vi "Handle Error.vi"(8 "error in (no error)":errorcluster, 11 "Entry Console API in":refnum<class "Entry Console API.lvclass">) -> (0 "error out":errorcluster, 2 "stop actor?":bool=TRUE, 3 "Entry Console API out":refnum<class "Entry Console API.lvclass">)   [LabVIEW 2012, in "Entry Console API.lvlib" / "Entry Console API.lvclass"]
doc: "(<B>Filename</B>: Actor Framework.lvlib:Actor.lvclass:Handle Error.vi)\n\nDefines how the actor handles an error that occurred while processing a message.\n\nBy default, this method does nothing except stop the actor. This method also treats error code 43 (coming from <B>error in</B>) as a sign that the actor shut down normally. In this situation, the Handle Error method does not return the error on <B>error out</B>, meaning the actor's caller will not receive it. All other error codes will be returned on <B>error out</B>.\n\nA descendant class may override this method to change this behavior."
uses:
  Entry Console API.lvclass
  <vilib>/ActorFramework/Actor/Actor.lvclass
  Car Wash Controller/Car Wash Controller Messages/Handle Nested Actor Error Msg/Handle Nested Actor Error Msg.lvclass
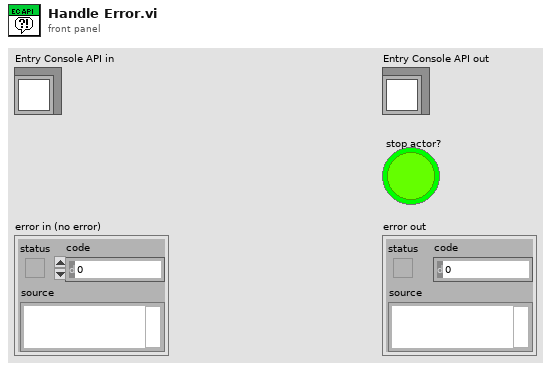
[diagram p1: front panel]
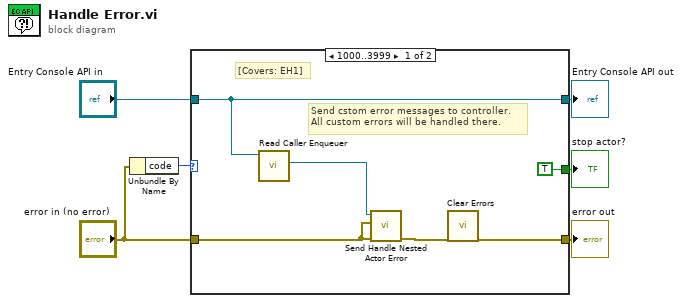
[diagram p0: block diagram]
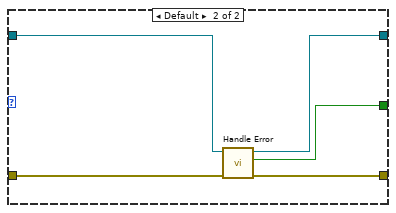
[diagram p2: hidden frame]
diagram:
  n1 = Unbundle By Name("error in (no error)") -> ("code"=w1:i32)
  n2 = case shown="1000..3999" w1 {
    tunnel: [w12 w17] -> w6
    tunnel: [TRUE ("stop actor?") w16] -> w5
    tunnel: [w9 w15] -> w4
    tunnel: "error in (no error)" -> [w10 w14]
    tunnel: "Entry Console API in" -> [w9 w13]
    frame 1000..3999 {
      # "Send cstom error messages to controller.\nAll custom errors will be handled there."
      # "[Covers: EH1]"
      n3 = call <vilib>:"Read Caller Enqueuer.vi"("Actor"=w9) -> ("Caller Enqueuer"=w8:refnum<class "Message Enqueuer.lvclass">)  [unwired: 10 in]
      n4 = call "Send Handle Nested Actor Error.vi"("error in (no error)"=w10, "Nested Actor Error"=w10, "Message Enqueuer"=w8) -> ("error out"=w11:errorcluster)  [unwired: 7 in, 1 out]
      n5 = call <vilib>:"Clear Errors.vi"("error in (no error)"=w11) -> ("error out"=w12:errorcluster)  [unwired: 5 in, 1 out]
    }
    frame Default {
      n6 = call-parent "Handle Error.vi"("error in (no error)"=w14, "Actor in"=w13) -> ("error out"=w17:errorcluster, "stop actor?"=w16:bool, "Actor out"=w15:refnum<class "Entry Console API.lvclass">)  [unwired: 7 in]
    }
  }
  "Entry Console API out" <- w4
  "error out" <- w6
  "stop actor?" <- w5
